vi "Register Events.vi"(8 "error in (no error)":errorcluster, 11 "Controller in":refnum<class "Controller.lvclass">) -> (0 "error out":errorcluster, 2 "Event Registration Refnum":refnum<event-registration>, 3 "Controller out":refnum<class "Controller.lvclass">)   [LabVIEW 2020, in "Controller.lvclass"]
uses:
  Controller.lvclass
  controls/Module response.ctl
  Controller.lvclass/Controller.ctl
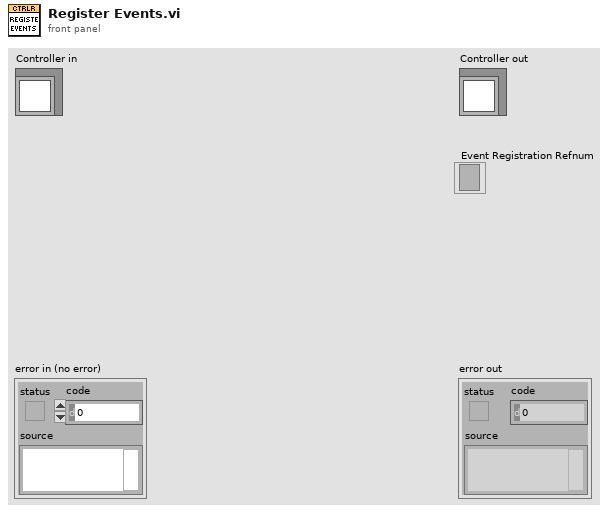
[diagram p1: front panel]
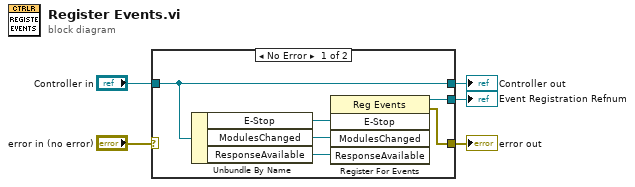
[diagram p0: block diagram]
diagram:
  n1 = case shown="No Error" "error in (no error)" {
    selector: "error in (no error)" -> [_ w13]
    tunnel: [w10 w13] -> w4
    tunnel: [w9 w12] -> w2
    tunnel: "Controller in" -> [w9 w12]
    tunnel: [w11 _] -> w1
    frame No Error {
      n2 = Unbundle By Name(w9) -> ("E-Stop"=w8:refnum<user-event>, "ModulesChanged"=w7:refnum<user-event>, "ResponseAvailable"=w6:refnum<user-event>)
      n3 = register-events(w8, w7, w6) -> (reference out=w11:refnum<event-registration>, error out=w10:errorcluster)  [unwired: 2 in]
    }
    frame Error {
    }
  }
  "error out" <- w4
  "Controller out" <- w2
  "Event Registration Refnum" <- w1
